vi "Draw Bone.vi"(7 "Joints":refnum<k24>, 8 "error in":errorcluster, 9 "Ending Joint":i32(ring)=2 items=["SpineBase", "SpineMid", "Neck", "Head", "ShoulderLeft", "ElbowLeft", "WristLeft", "HandLeft", "ShoulderRight", "ElbowRight", "WristRight", "HandRight", "HipLeft", "KneeLeft", "AnkleLeft", "FootLeft", "HipRight", "KneeRight", "AnkleRight", "FootRight", "SpineShoulder", "HandTipLeft", "ThumbLeft", "HandTipRight", "ThumbRight"], 10 "Starting Joint":i32(ring)=3 items=["SpineBase", "SpineMid", "Neck", "Head", "ShoulderLeft", "ElbowLeft", "WristLeft", "HandLeft", "ShoulderRight", "ElbowRight", "WristRight", "HandRight", "HipLeft", "KneeLeft", "AnkleLeft", "FootLeft", "HipRight", "KneeRight", "AnkleRight", "FootRight", "SpineShoulder", "HandTipLeft", "ThumbLeft", "HandTipRight", "ThumbRight"], 11 "Image":T1) -> (0 "error out":errorcluster, 3 "Image Out":T1)   [LabVIEW 2014]
uses:
  <vilib>/vision/Image Controls.llb/IMAQ Image.ctl
  Microsoft.Kinect
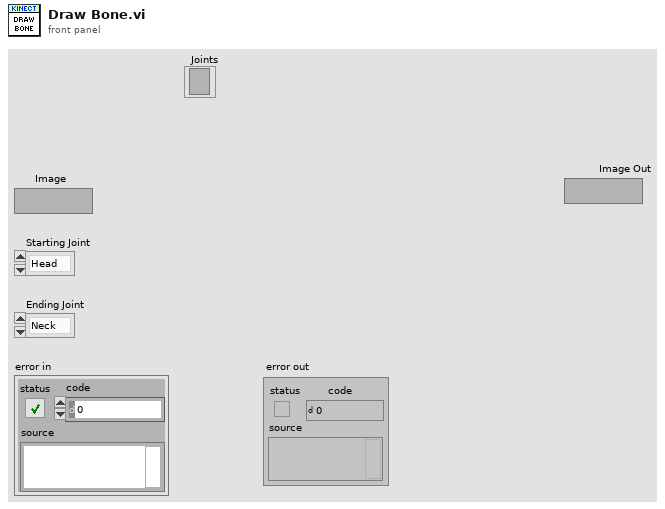
[diagram p1: front panel]
types:
  T1 = typedef "IMAQ Image.ctl" = refnum<image>
  T2 = enum16{"Get Attribute", "Initialize", "Set Attribute"}
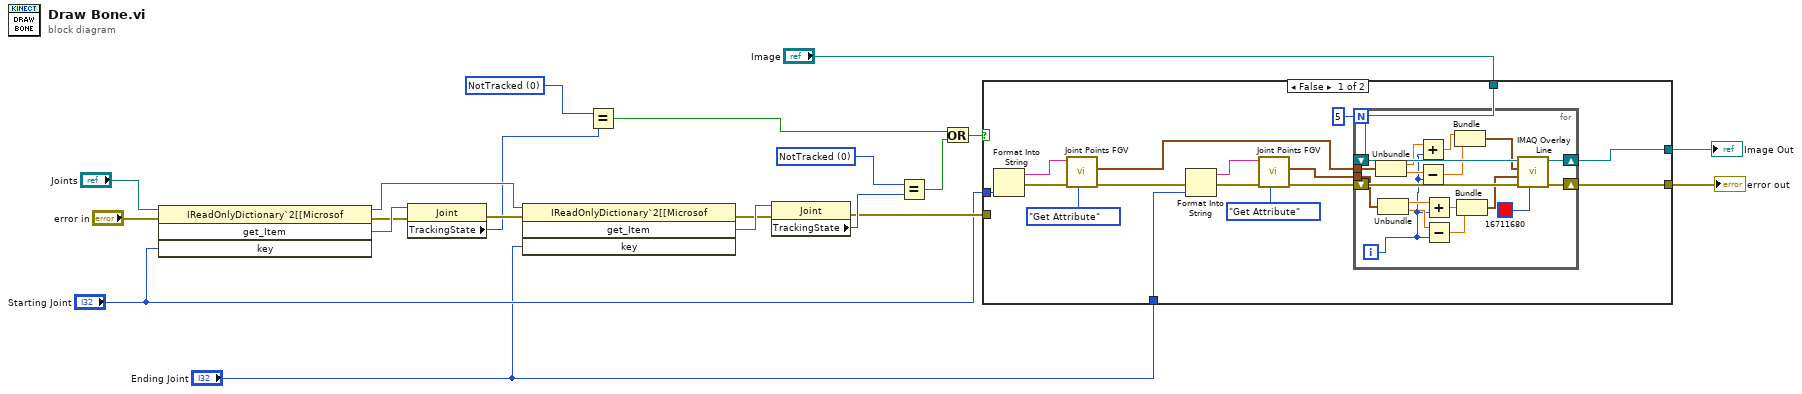
[diagram p0: block diagram]
diagram:
  w9 = 0 items=["NotTracked", "Inferred", "Tracked"] ("TrackingState")
  w11 = 0 items=["NotTracked", "Inferred", "Tracked"] ("TrackingState")
  n1 = invoke class="IReadOnlyDictionary`2[[Microsof" method="get_Item"(reference="Joints", error in="error in", "key"="Starting Joint") -> (reference out=w12:refnum<k24>, error out=w16:errorcluster, "get_Item"=w17:refnum<k24>)  [unwired: 1 in, 1 out]
  n2 = property class="Joint"(reference=w17, error in=w16) -> (error out=w13:errorcluster, "TrackingState"=w10:i32)  [unwired: 1 out]
  n3 = invoke class="IReadOnlyDictionary`2[[Microsof" method="get_Item"(reference=w12, error in=w13, "key"="Ending Joint") -> (error out=w14:errorcluster, "get_Item"=w15:refnum<k24>)  [unwired: 1 in, 2 out]
  n4 = Equal?(x=w11, y=w10) -> (x = y?=w5:bool)
  n5 = property class="Joint"(reference=w15, error in=w14) -> (error out=w4:errorcluster, "TrackingState"=w8:i32)  [unwired: 1 out]
  n6 = Equal?(x=w9, y=w8) -> (x = y?=w6:bool)
  n7 = Or(x=w5, y=w6) -> (x .or. y?=w7:bool)
  n8 = case shown="False" w7 {
    tunnel: "Starting Joint" -> [w36 _]
    tunnel: "Ending Joint" -> [w32 _]
    tunnel: "Image" -> [w25 w56]
    tunnel: [w24 w57] -> w20
    tunnel: [w23 w56] -> w19
    tunnel: w4 -> [_ w57]
    frame False {
      n9 = Format Into String(w36) -> (resulting string=w35:string, error out=w34:errorcluster)  [unwired: 3 in]
      n10 = call "Joint Points FGV.vi"("Command"=T2."Get Attribute", "error in (no error)"=w34, "name"=w35) -> ("error out"=w31:errorcluster, "Joint Point"=w27:cluster{"X":sgl, "Y":sgl})  [unwired: 7 in]
      n11 = Format Into String(error in=w31, w32) -> (resulting string=w30:string, error out=w33:errorcluster)  [unwired: 2 in]
      n12 = call "Joint Points FGV.vi"("Command"=T2."Get Attribute", "error in (no error)"=w33, "name"=w30) -> ("error out"=w28:errorcluster, "Joint Point"=w26:cluster{"X":sgl, "Y":sgl})  [unwired: 7 in]
      n13 = for {
        N: 5 -> [_]
        tunnel: w27 -> [w50]
        tunnel: w26 -> [w49]
        shift-right: [w53] -> w24
        shift-left: w28 -> [w55]
        shift-right: [w52] -> w23
        shift-left: w25 -> [w54]
        i -> [w44]
        n14 = Unbundle(w50) -> ("X"=w45:sgl, "Y"=w46:sgl)
        n15 = Unbundle(w49) -> ("X"=w48:sgl, "Y"=w47:sgl)
        n16 = Add(x=w45, y=w44) -> (x+y=w43:sgl)
        n17 = Subtract(x=w46, y=w44) -> (x-y=w42:sgl)
        n18 = Add(x=w48, y=w44) -> (x+y=w40:sgl)
        n19 = Subtract(x=w47, y=w44) -> (x-y=w39:sgl)
        n20 = Bundle(w43, w42) -> (w41:cluster{sgl, sgl})  [unwired: 1 in]
        n21 = Bundle(w40, w39) -> (w38:cluster{sgl, sgl})  [unwired: 1 in]
        n22 = call "IMAQ Overlay Line"("Color"=u32 16711680, "error in (no error)"=w55, "End Point"=w38, "Start Point"=w41, "Image"=w54) -> ("error out"=w53:errorcluster, "Image Out"=w52:T1)  [unwired: 5 in]
      }
    }
    frame True {
    }
  }
  "error out" <- w20
  "Image Out" <- w19
